vi "Read executiontime.vi"(8 "error in (no error)":errorcluster, 11 "syslogs in":refnum<class "syslogs.lvclass">) -> (0 "error out":errorcluster, 2 "executiontime":dbl, 3 "syslogs out":refnum<class "syslogs.lvclass">)   [LabVIEW 2020, in "ORM_Examples.lvlib" / "syslogs.lvclass"]
uses:
  syslogs.lvclass
  syslogs.lvclass/syslogs.ctl
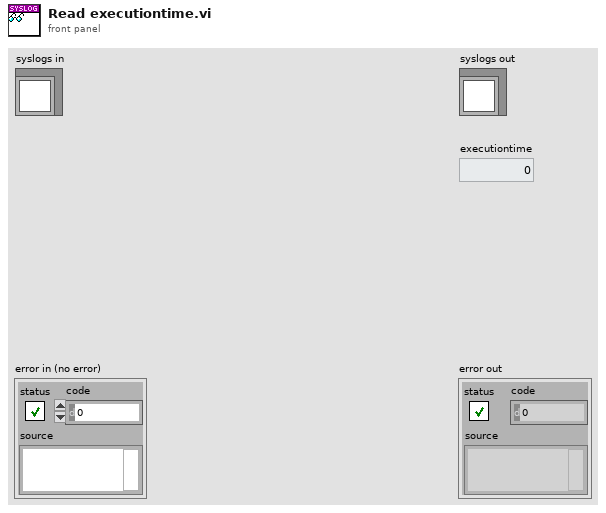
[diagram p1: front panel]
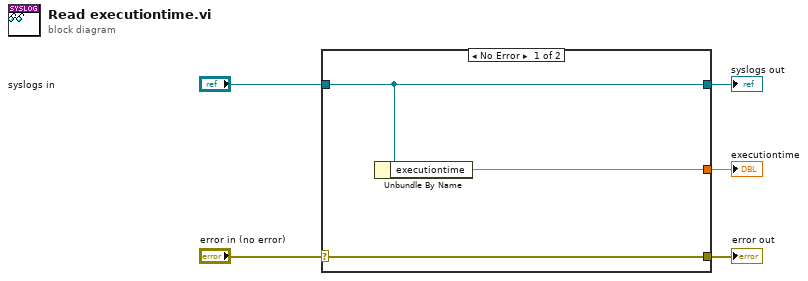
[diagram p0: block diagram]
diagram:
  n1 = case shown="No Error" "error in (no error)" {
    selector: "error in (no error)" -> [w8 w9]
    tunnel: [w8 w9] -> w4
    tunnel: [w7 w10] -> w2
    tunnel: "syslogs in" -> [w7 w10]
    tunnel: [w6 _] -> w1
    frame No Error {
      n2 = Unbundle By Name(w7) -> ("executiontime"=w6:dbl)
    }
    frame Error {
    }
  }
  "error out" <- w4
  "syslogs out" <- w2
  "executiontime" <- w1
